vi "Master Setup Titles.vi"() -> (0 "Sorted Titles Indices":i32[](array[numeric]), 1 "Setup Patterns":string[](array[string]), 2 "Setup Description":string[](array[string]), 3 "Setup Description w/Numbers":string[](array[string]), 4 "Sorted Setup Description":string[](array[string]), 6 "Sorted Setup Patterns":string[](array[string]))   [LabVIEW 2017]
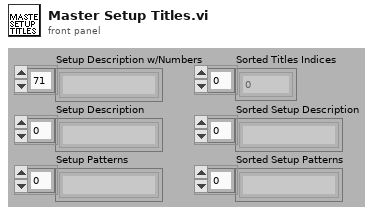
[diagram p1: front panel]
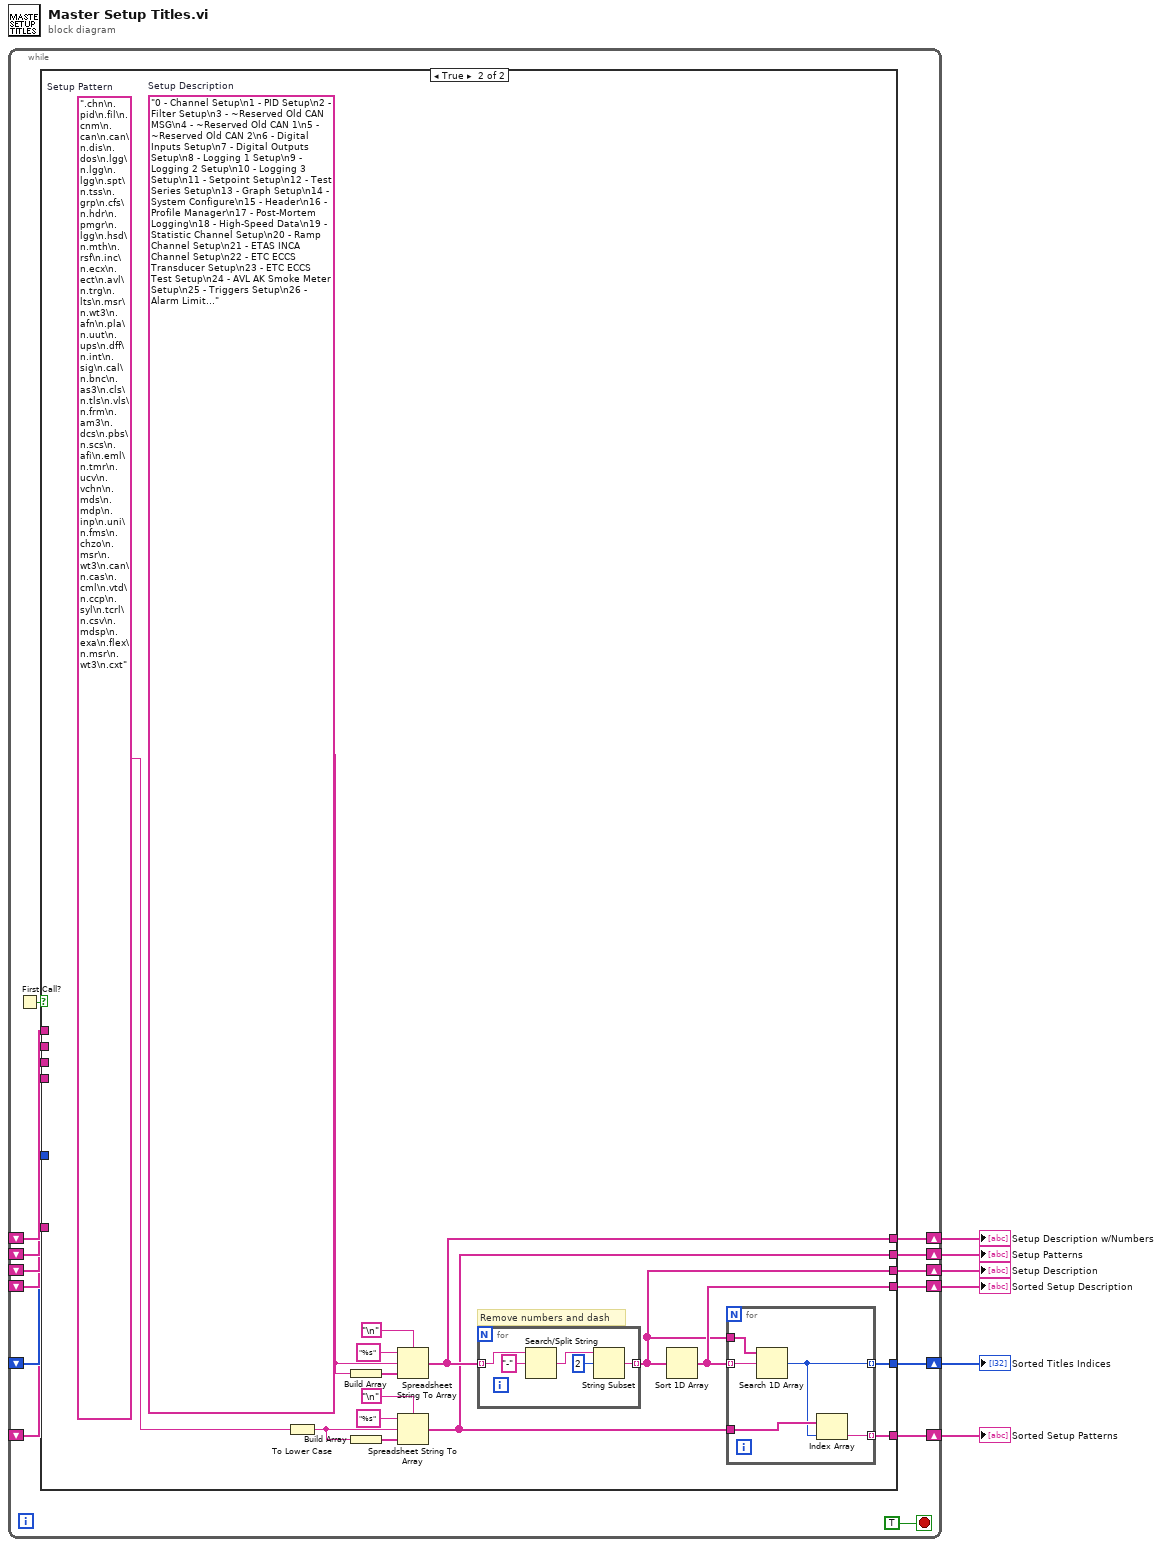
[diagram p0: block diagram]
diagram:
  n1 = while {
    shift-right: [w20] -> w6
    shift-left: _ -> [w13]
    shift-right: [w17] -> w3
    shift-left: _ -> [w12]
    shift-right: [w18] -> w4
    shift-left: _ -> [w11]
    shift-right: [w19] -> w5
    shift-left: _ -> [w10]
    shift-right: [w16] -> w2
    shift-left: _ -> [w9]
    shift-right: [w15] -> w1
    shift-left: _ -> [w8]
    stop <- TRUE stop-if-true
    n2 = First Call?() -> (First Call?: T/F=w14:bool)
    n3 = case shown="True" w14 {
      tunnel: [w26 w40] -> w20
      tunnel: [w23 w32] -> w19
      tunnel: [w24 w31] -> w18
      tunnel: [w25 w30] -> w17
      tunnel: [w22 w29] -> w16
      tunnel: [w21 w28] -> w15
      tunnel: w13 -> [w26 _]
      tunnel: w12 -> [w25 _]
      tunnel: w11 -> [w24 _]
      tunnel: w10 -> [w23 _]
      tunnel: w9 -> [w22 _]
      tunnel: w8 -> [w21 _]
      frame False {
      }
      frame True {
        w39 = ".chn\n.pid\n.fil\n.cnm\n.can\n.can\n.dis\n.dos\n.lgg\n.lgg\n.lgg\n.spt\n.tss\n.grp\n.cfs\n.hdr\n.pmgr\n.lgg\n.hsd\n.mth\n.rsf\n.inc\n.ecx\n.ect\n.avl\n.trg\n.lts\n.msr\n.wt3\n.afn\n.pla\n.uut\n.ups\n.dff\n.int\n.sig\n.cal\n.bnc\n.as3\n.cls\n.tls\n.vls\n.frm\n.am3\n.dcs\n.pbs\n.scs\n.afi\n.eml\n.tmr\n.ucv\n.vchn\n.mds\n.mdp\n.inp\n.uni\n.fms\n.chzo\n.msr\n.wt3\n.can\n.cas\n.cml\n.vtd\n.ccp\n.syl\n.tcrl\n.csv\n.mdsp\n.exa\n.flex\n.msr\n.wt3\n.cxt"  # Setup Pattern
        w33 = "0 - Channel Setup\n1 - PID Setup\n2 - Filter Setup\n3 - ~Reserved Old CAN MSG\n4 - ~Reserved Old CAN 1\n5 - ~Reserved Old CAN 2\n6 - Digital Inputs Setup\n7 - Digital Outputs Setup\n8 - Logging 1 Setup\n9 - Logging 2 Setup\n10 - Logging 3 Setup\n11 - Setpoint Setup\n12 - Test Series Setup\n13 - Graph Setup\n14 - System Configure\n15 - Header\n16 - Profile Manager\n17 - Post-Mortem Logging\n18 - High-Speed Data\n19 - Statistic Channel Setup\n20 - Ramp Channel Setup\n21 - ETAS INCA Channel Setup\n22 - ETC ECCS Transducer Setup\n23 - ETC ECCS Test Setup\n24 - AVL AK Smoke Meter Setup\n25 - Triggers Setup\n26 - Alarm Limits Setup\n27 - YKWT1 Measurement\n28 - YKWT1 Instrument\n29 - Auto File Settings\n30 - Playback File Setting\n31 - UUT Constants\n32 - UPS Setup\n33 - Differential Channel Setup\n34 - Integral Channel Setup\n35 - Signal Channel Setup\n36 - Calibration Setup\n37 - BNC Setup\n38 - ASAP3 Setup\n39 - Chassis Force Calculations\n40 - Chassis Teststand Losses\n41 - Chassis Vehicle Losses\n42 - Formula Channels\n43 - ASAP3 Map Coords Setup\n44 - Digital Controls Setup\n45 - Push Buttons Setup\n46 - Sliders Setup\n47 - ~Reserved~\n48 - Email Setup\n49 - Timer Setup\n50 - Unit Conversion Setup\n51 - Visible Channels\n52 - Main Display Setup\n53 - Message Display Setup\n54 - Input Display Setup\n55 - Unico Parameter Downloads\n56 - Flow Meter Setup\n57 - Channel Zero Offset\n58 - YKWT2 Measurement\n59 - YKWT2 Instrument\n60 - ~Reserved Old CAN 3\n61 - CAS Setup\n62 - Accumulation Channel Setup\n63 - Valvetrain Dynamics Setup\n64 - CCP Setup\n65 - System Log Setup\n66 - Throttle Controller\n67 - RE Shifter\n68 - Main Display\n69 - ~Reserved~\n70 - FlexRay\n71 - YKWT3 Measurement\n72 - YKWT3 Instrument\n73 - CAN XNET API"  # Setup Description
        # "Remove numbers and dash"
        n4 = To Lower Case(string=w39) -> (all lower case string=w41:string)
        n5 = Build Array(w33) -> (w34:string[])
        n6 = Build Array(w41) -> (w38:string[])
        n7 = Spreadsheet String To Array(delimiter (Tab)="\n", format string="%s", spreadsheet string=w33, array type (2D Dbl)=w34) -> (array=w40:string[])
        n8 = Spreadsheet String To Array(delimiter (Tab)="\n", format string="%s", spreadsheet string=w41, array type (2D Dbl)=w38) -> (array=w30:string[])
        n9 = for {
          tunnel: w40 -> [w51] mode=indexing
          tunnel: [w47] -> w31 mode=indexing
          n10 = Search/Split String(string=w51, search string/char (-)="-") -> (match + rest of string=w49:string)  [unwired: 1 in, 2 out]
          n11 = String Subset(string=w49, offset (0)=2) -> (substring=w47:string)  [unwired: 1 in]
        }
        n12 = Sort 1D Array(array=w31) -> (sorted array=w32:string[])
        n13 = for {
          tunnel: w32 -> [w45] mode=indexing
          tunnel: w31 -> [w46]
          tunnel: [w43] -> w29 mode=indexing
          tunnel: w30 -> [w44]
          tunnel: [w42] -> w28 mode=indexing
          n14 = Search 1D Array(1D array=w46, element=w45) -> (index of element=w43:i32)  [unwired: 1 in]
          n15 = Index Array(array=w44, index=w43) -> (element=w42:string)
        }
      }
    }
  }
  "Setup Description" <- w4
  "Setup Description w/Numbers" <- w6
  "Setup Patterns" <- w3
  "Sorted Setup Description" <- w5
  "Sorted Titles Indices" <- w2
  "Sorted Setup Patterns" <- w1
